vi "GetRidOf66.vi"(1 "error in (no error)":errorcluster) -> (0 "error out":errorcluster)   [LabVIEW 2013]
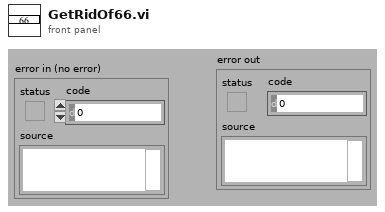
[diagram p1: front panel]
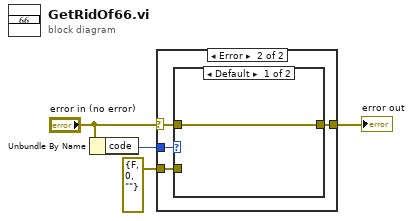
[diagram p0: block diagram]
diagram:
  n1 = Unbundle By Name("error in (no error)") -> ("code"=w2:i32)
  n2 = case shown="Error" "error in (no error)" {
    selector: "error in (no error)" -> [w5 w6]
    tunnel: [w5 w8] -> w4
    tunnel: w2 -> [_ w9]
    tunnel: errorcluster {"status"=FALSE, "code"=0, "source"=""} ("error in (no error)") -> [_ w7]
    frame No Error {
    }
    frame Error {
      n3 = case shown="Default" w9 {
        tunnel: [w10 w11] -> w8
        tunnel: w7 -> [_ w11]
        tunnel: w6 -> [w10 _]
        frame Default {
        }
        frame 66 {
        }
      }
    }
  }
  "error out" <- w4
